vi "4.SFTP.vi"() -> ()   [LabVIEW 2017]
uses:
  UnderAutomation.UniversalRobots/UnderAutomation.UniversalRobots.lvlib
  C:/Users/fg/Documents/UniversalRobots.vi/LabVIEW_2024/UnderAutomation.UniversalRobots/lib/UnderAutomation.UniversalRobots.dll
  LabVIEW_2024/UnderAutomation.UniversalRobots/lib/UnderAutomation.UniversalRobots.dll
panel:
  out "Sftp":refnum<k24>
  out "UR Robot":refnum<k24>
  out "Connected":bool
  in  "Tab Control":enum32{"Connect to robot", "SFTP"}(tab)
  in  "Username":string(combo)
  in  "Disconnect":bool
  in  "Test":bool
  in  "Key":string
  in  "Licensee":string
  in  "Connect":bool
  in  "IP":string caption="Robot IP Address"
  out "License state":string
  out "Connect error":string
  in  "Password":string
  in  "Local Path":path
  in  "Enumerate installations":bool
  out "Installations":string[](array[string])
  in  "Delete":bool
  in  "File or directory to delete":string
  in  "Upload":bool
  in  "Download":bool
  in  "Robot Path":string
  out "DirectoryItems":T1(array[cluster])
  in  "Directory to create":string
  in  "Create directory":bool
  in  "List directory":bool
  in  "Robot Path":string
  in  "Enumerate programs":bool
  out "Programs":string[](array[string])
  out "error out":errorcluster
  in  "stop":bool
  # "UnderAutomation"
  # "https://underautomation.com/universal-robots"
  # "+"
  # "LabVIEW demo app for remote control and monitoring of your Universal Robots cobot"
  # "Connect to robot"
  # "2. Ensure you have a trial or lifetime valid license"
  # "1. Set UR cobot address"
  # "This is a commercial library, you have a 30-day trial period. But you can use it forever if you buy a perpetual licence for your company (regardless of the number of robot, applications or developers)."
  # "If you have a license :"
  # "2. Set SSH access"
  # "Username is \"ur\" for simulator and \"root\" on a real robot"
  # "Default password is \"easybot\""
  # "3. Connect to the robot"
  # "Create directory"
  # "List directory"
  # "Upload and download"
  # "Delete"
  # "Installations"
  # "Programs"
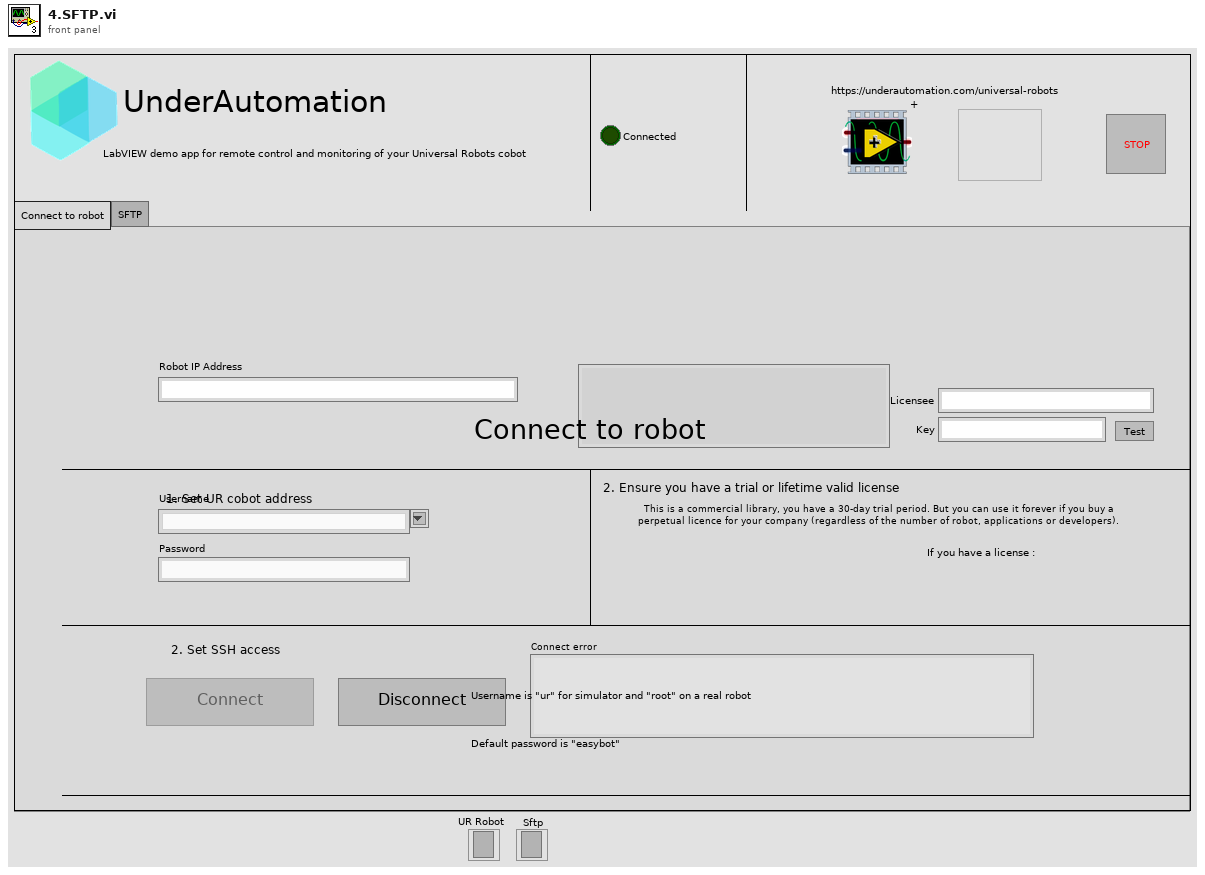
[diagram p1: front panel]
types:
  T1 = cluster{"Name":string, "FullName":string, "Length":i64, "IsDirectory":bool, "IsSymbolicLink":bool, "IsBlockDevice":bool, "IsCharacterDevice":bool, "IsNamedPipe":bool, "IsRegularFile":bool, "IsSocket":bool, "LastAccessTime":timestamp, "LastWriteTime":timestamp}[]
  T2 = enum8{"Enabled", "Disabled", "Disabled and Grayed Out"}
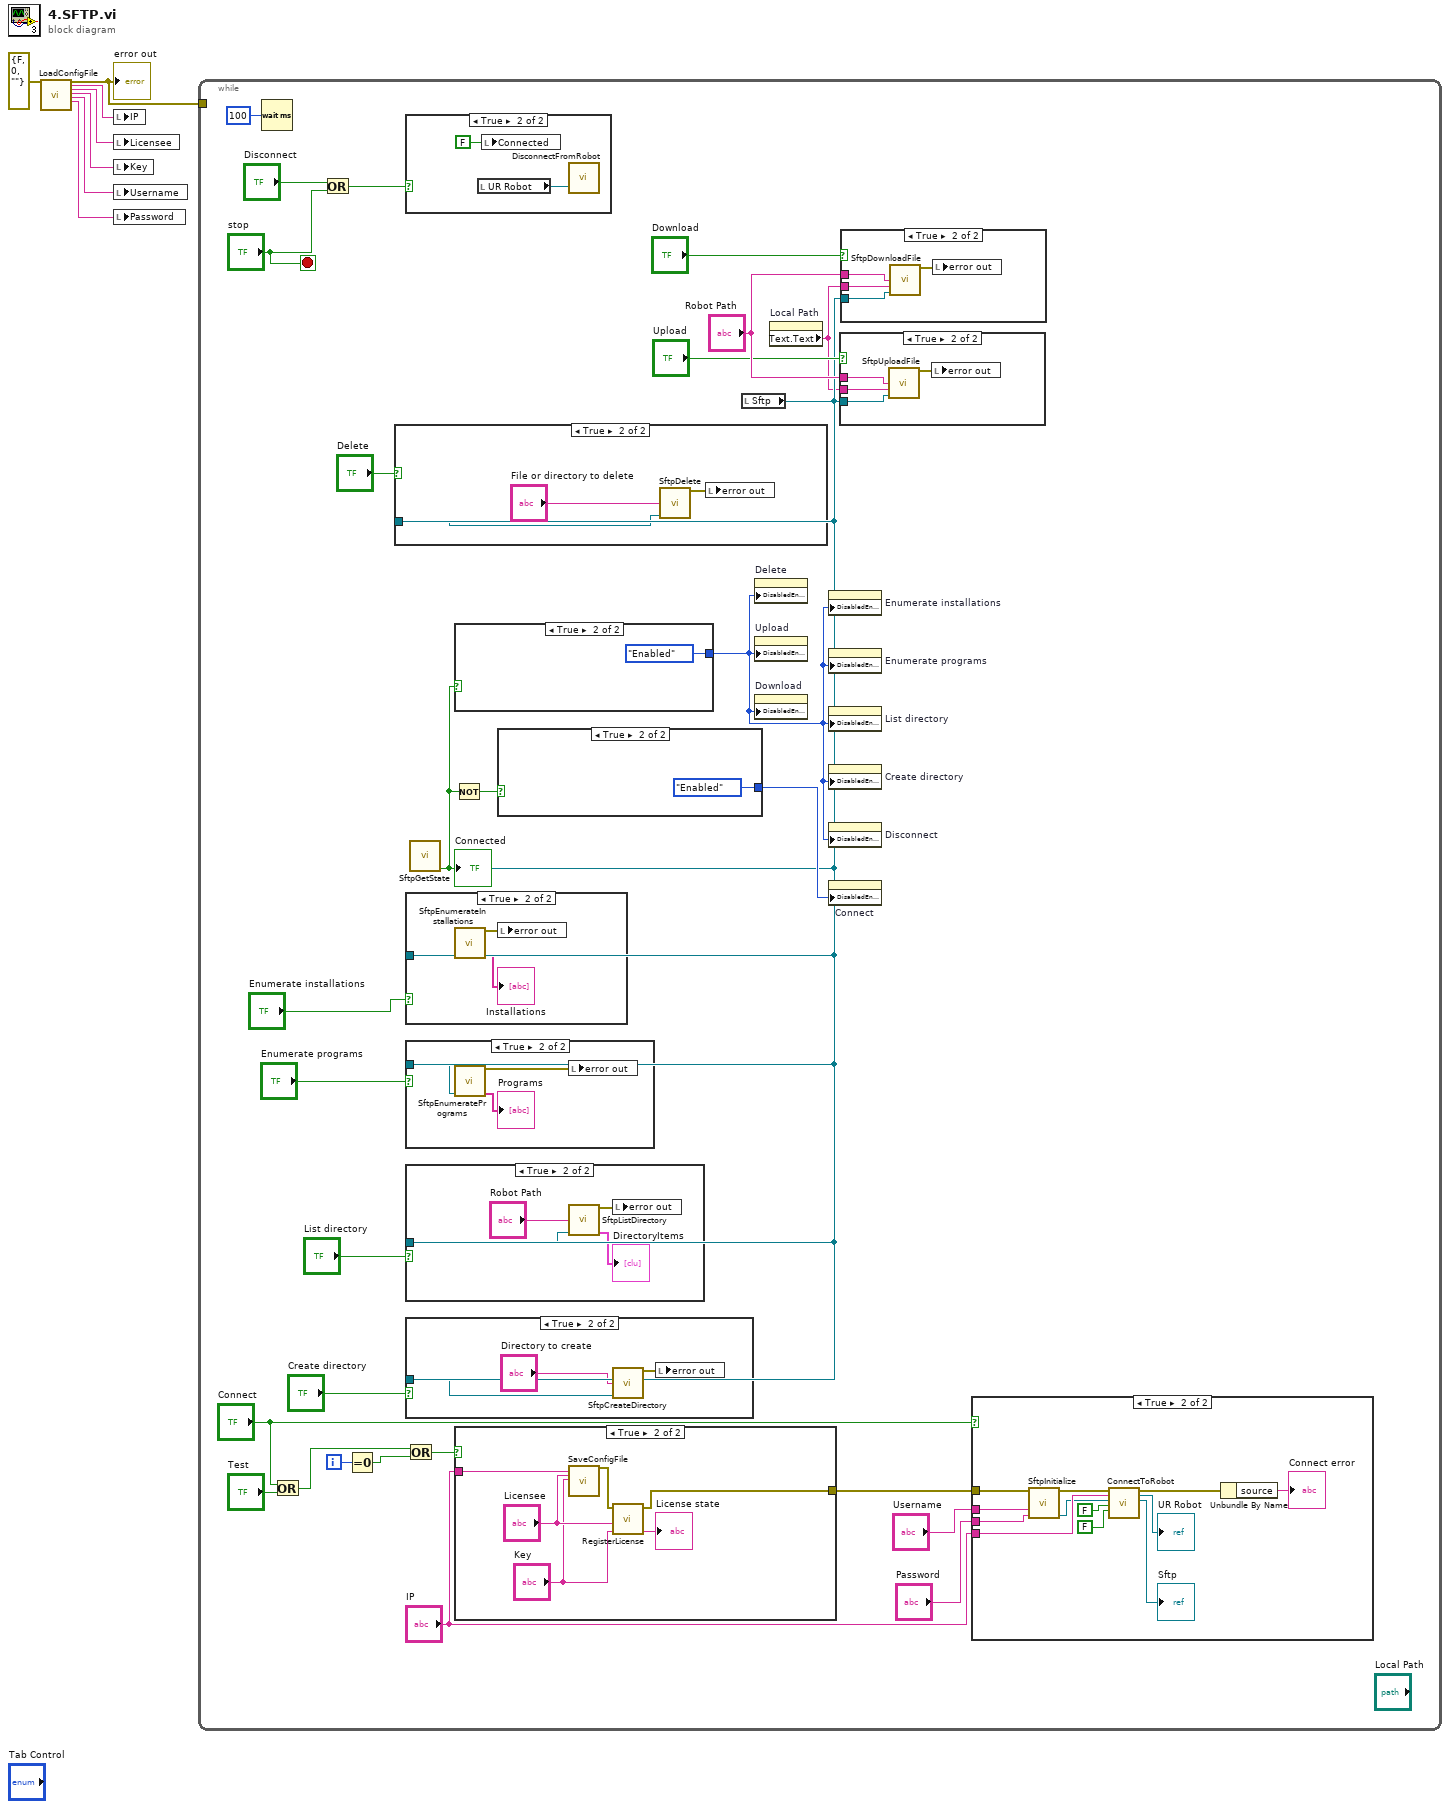
[diagram p0: block diagram]
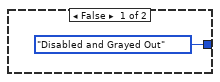
[diagram p9: hidden frame]
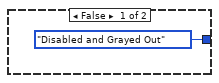
[diagram p10: hidden frame]
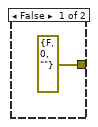
[diagram p11: hidden frame]
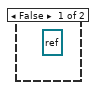
[diagram p12: hidden frame]
diagram:
  n1 = call "LoadConfigFile.vi"("error in (no error)"=errorcluster {"status"=FALSE, "code"=0, "source"=""}) -> ("error out"=w4:errorcluster, "IP"=w5:string, "Licensee"=w7:string, "Key"=w6:string, "Username"=w3:string, "Password"=w2:string)  [unwired: 21 in]
  "error out" <- w4
  n2 = local write "IP"(w5) -> ()
  n3 = local write "Licensee"(w7) -> ()
  n4 = local write "Key"(w6) -> ()
  n5 = local write "Username"(w3) -> ()
  n6 = local write "Password"(w2) -> ()
  n7 = while {
    tunnel: w4 -> [_]
    i -> [w29]
    stop <- "stop" stop-if-true
    n8 = Wait (ms)(milliseconds to wait=u32 100) -> ()  [unwired: 1 out]
    n9 = Or(x="Connect", y="Test") -> (x .or. y?=w27:bool)
    n10 = Or(x="Disconnect", y="stop") -> (x .or. y?=w33:bool)
    n11 = Equal To 0?(x=w29) -> (x = 0?=w28:bool)
    n12 = case shown="True" w33 {
      frame False {
      }
      frame True {
        n13 = local read "UR Robot"() -> (w84:refnum<k24>)
        n14 = local write "Connected"(FALSE ("Connected")) -> ()
        n15 = call "DisconnectFromRobot.vi"("UR Robot"=w84) -> ()  [unwired: 2 in, 1 out]
      }
    }
    n16 = Or(x=w27, y=w28) -> (x .or. y?=w26:bool)
    n17 = case shown="True" w26 {
      tunnel: [errorcluster {"status"=FALSE, "code"=0, "source"=""} ("error out") w69] -> w25
      tunnel: "IP" -> [_ w66]
      frame False {
      }
      frame True {
        n18 = call "SaveConfigFile.vi"("IP"=w66, "Licensee"="Licensee", "Key"="Key") -> ("error out"=w65:errorcluster)  [unwired: 24 in]
        n19 = call "RegisterLicense.vi"("key"="Key", "licensee"="Licensee", "error in"=w65) -> ("State message"=→"License state":string, "error out"=w69:errorcluster)  [unwired: 5 in, 1 out]
      }
    }
    n20 = local read "Sftp"() -> (w11:refnum<k24>)
    n21 = case shown="True" "Delete" {
      tunnel: w11 -> [_ w43]
      frame False {
      }
      frame True {
        n22 = call "SftpDelete.vi"("Robot Path"="File or directory to delete", "Sftp"=w43) -> ("error out"=w42:errorcluster)  [unwired: 13 in]
        n23 = local write "error out"(w42) -> ()
      }
    }
    n24 = case shown="True" "Enumerate installations" {
      tunnel: w11 -> [_ w59]
      frame False {
      }
      frame True {
        n25 = call "SftpEnumerateInstallations.vi"("Sftp"=w59) -> ("error out"=w57:errorcluster, "Installations"=→"Installations":string[])  [unwired: 13 in]
        n26 = local write "error out"(w57) -> ()
      }
    }
    n27 = case shown="True" "Enumerate programs" {
      tunnel: w11 -> [_ w37]
      frame False {
      }
      frame True {
        n28 = call "SftpEnumeratePrograms.vi"("Sftp"=w37) -> ("error out"=w36:errorcluster, "Programs"=→"Programs":string[])  [unwired: 13 in]
        n29 = local write "error out"(w36) -> ()
      }
    }
    n30 = case shown="True" "List directory" {
      tunnel: w11 -> [_ w55]
      frame False {
      }
      frame True {
        n31 = call "SftpListDirectory.vi"("Robot Path"="Robot Path", "Sftp"=w55) -> ("error out"=w53:errorcluster, "DirectoryItems"=→"DirectoryItems":T1)  [unwired: 12 in]
        n32 = local write "error out"(w53) -> ()
      }
    }
    n33 = case shown="True" "Create directory" {
      tunnel: w11 -> [_ w41]
      frame False {
      }
      frame True {
        n34 = call "SftpCreateDirectory.vi"("Robot Path"="Directory to create", "Sftp"=w41) -> ("error out"=w39:errorcluster)  [unwired: 13 in]
        n35 = local write "error out"(w39) -> ()
      }
    }
    n36 = call "SftpGetState.vi"("Sftp"=w11) -> ("Connected"=w19:bool)  [unwired: 13 in, 1 out]
    "Connected" <- w19
    n37 = Not(x=w19) -> (.not. x?=w23:bool)
    n38 = case shown="True" w19 {
      tunnel: [T2."Disabled and Grayed Out" ("Disabled") T2."Enabled" ("Disabled")] -> w8
      frame False {
      }
      frame True {
      }
    }
    n39 = case shown="True" w23 {
      tunnel: [T2."Disabled and Grayed Out" ("Disabled") T2."Enabled" ("Disabled")] -> w22
      frame False {
      }
      frame True {
      }
    }
    n40 = property on="Delete" class="Bool"("DisabledEnum"=w8) -> ()  [unwired: 2 in, 2 out]
    n41 = property on="Upload" class="Bool"("DisabledEnum"=w8) -> ()  [unwired: 2 in, 2 out]
    n42 = property on="Download" class="Bool"("DisabledEnum"=w8) -> ()  [unwired: 2 in, 2 out]
    n43 = property on="Local Path" class="Path"() -> ("Text.Text"=w9:string)  [unwired: 2 in, 2 out]
    n44 = property on="Enumerate installations" class="Bool"("DisabledEnum"=w8) -> ()  [unwired: 2 in, 2 out]
    n45 = property on="Enumerate programs" class="Bool"("DisabledEnum"=w8) -> ()  [unwired: 2 in, 2 out]
    n46 = property on="List directory" class="Bool"("DisabledEnum"=w8) -> ()  [unwired: 2 in, 2 out]
    n47 = property on="Create directory" class="Bool"("DisabledEnum"=w8) -> ()  [unwired: 2 in, 2 out]
    n48 = property on="Disconnect" class="Bool"("DisabledEnum"=w8) -> ()  [unwired: 2 in, 2 out]
    n49 = property on="Connect" class="Bool"("DisabledEnum"=w22) -> ()  [unwired: 2 in, 2 out]
    n50 = case shown="True" "Upload" {
      tunnel: "Robot Path" -> [_ w48]
      tunnel: w9 -> [_ w47]
      tunnel: w11 -> [_ w46]
      frame False {
      }
      frame True {
        n51 = call "SftpUploadFile.vi"("Robot Path"=w48, "Local Path"=w47, "Sftp"=w46) -> ("error out"=w45:errorcluster)  [unwired: 12 in]
        n52 = local write "error out"(w45) -> ()
      }
    }
    n53 = case shown="True" "Download" {
      tunnel: w11 -> [_ w52]
      tunnel: "Robot Path" -> [_ w51]
      tunnel: w9 -> [_ w50]
      frame False {
      }
      frame True {
        n54 = call "SftpDownloadFile.vi"("Robot Path"=w51, "Local Path"=w50, "Sftp"=w52) -> ("error out"=w49:errorcluster)  [unwired: 12 in]
        n55 = local write "error out"(w49) -> ()
      }
    }
    n56 = case shown="True" "Connect" {
      tunnel: w25 -> [_ w75]
      tunnel: "IP" -> [_ w79]
      tunnel: "Password" -> [_ w72]
      tunnel: "Username" -> [_ w71]
      frame False {
        (unwired) refnum<k24> refnum ("Dashboard")
      }
      frame True {
        n57 = call "SftpInitialize.vi"("error in"=w75, "Username"=w71, "Password"=w72) -> ("error out"=w74:errorcluster, "SFTP Connect Parameters"=w73:refnum<k24>)  [unwired: 11 in]
        n58 = call "ConnectToRobot.vi"("error in"=w74, "ip"=w79, "SFTP Connect Parameters"=w73, "Enable Dashboard"=FALSE ("Enable Primary Interface"), "Enable Primary Interface"=FALSE) -> ("error out"=w82:errorcluster, "UR Robot"=→"UR Robot":refnum<k24>, "Sftp"=→"Sftp":refnum<k24>)  [unwired: 9 in, 3 out]
        n59 = Unbundle By Name(w82) -> ("source"=→"Connect error":string)
      }
    }
  }
